vi "Get Digital IO Pins Mode.vi"(8 "error in (no error)":errorcluster, 10 "Digital IO Line (1)":u32=1, 11 "VISA resource name":refnum<visa-resource-name>) -> (0 "error out":errorcluster, 2 "Digital I/O State?":string, 3 "VISA resource name out":refnum<visa-resource-name>)   [LabVIEW 2021, in "Keithley 2450.lvlib"]
doc: "Gets the digital I/O line state of the selected line."
uses:
  <instrlib>/Keithley 2450/Keithley 2450.lvlib
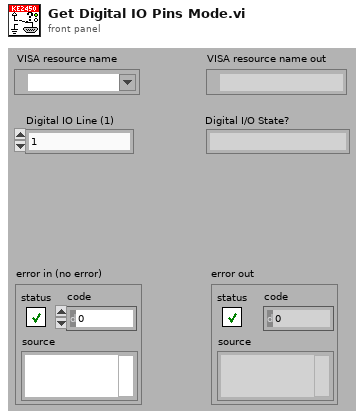
[diagram p1: front panel]
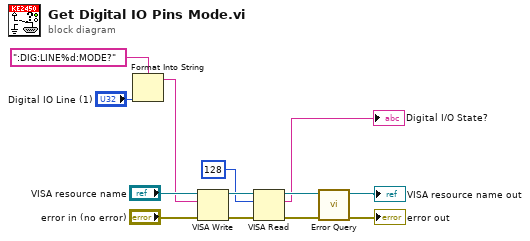
[diagram p0: block diagram]
diagram:
  n1 = Format Into String(format string=":DIG:LINE%d:MODE?", "Digital IO Line (1)") -> (resulting string=w7:string)  [unwired: 2 in, 1 out]
  n2 = VISA Write(VISA resource name="VISA resource name", write buffer=w7, error in (no error)="error in (no error)") -> (VISA resource name out=w6:refnum<visa-resource-name>, error out=w5:errorcluster)  [unwired: 1 out]
  n3 = VISA Read(VISA resource name=w6, byte count=u32 128, error in (no error)=w5) -> (VISA resource name out=w3:refnum<visa-resource-name>, read buffer=→"Digital I/O State?":string, error out=w4:errorcluster)  [unwired: 1 out]
  n4 = call <instrlib>:"Error Query.vi"("error in (no error)"=w4, "VISA resource name"=w3) -> ("error out"=→"error out":errorcluster, "VISA resource name out"=→"VISA resource name out":refnum<visa-resource-name>)  [unwired: 8 out]
